vi "BRig_dataCurrent_T_Cue2.vi"() -> (2 "output_T_Cue2":i32)   [LabVIEW 2014]
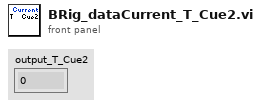
[diagram p1: front panel]
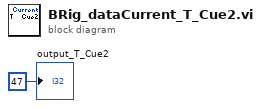
[diagram p0: block diagram]
diagram:
  "output_T_Cue2" <- 47 ("output_iBlock")
